vi "DB_Execute_Query.vi"() -> ()   [LabVIEW 2020]
uses:
  <vilib>/addons/database/Connection.llb/DB Tools Open Connec (String).vi
  <vilib>/addons/database/Connection.llb/Conn Execute.vi
  <vilib>/addons/database/Recordset.llb/Rec Fetch Recordset Data (R).vi
  <vilib>/addons/database/Recordset.llb/Rec Destroy - Connection.vi
  <vilib>/addons/database/NI_Database_API.lvlib
panel:
  out "recordset data":variant[][](array[variant])
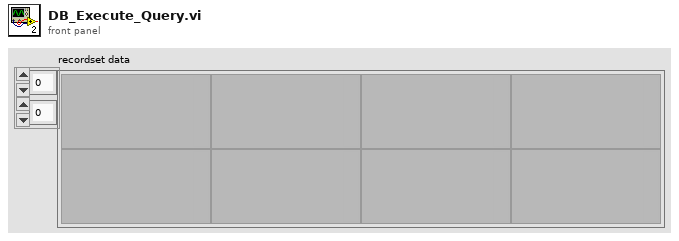
[diagram p1: front panel]
types:
  T1 = typedef "NI_Database_API.lvlib/Conn ObjectReference.ctl" = refnum<k1>
  T2 = typedef "NI_Database_API.lvlib/Rec ObjectReference.ctl" = refnum<k1>
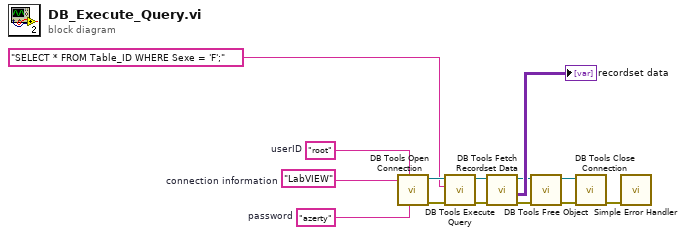
[diagram p0: block diagram]
diagram:
  w2 = "azerty"  # password
  w3 = "root"  # userID
  w4 = "LabVIEW"  # connection information
  n1 = call-poly <vilib>:"DB Tools Open Connection.vi"("password"=w2, "userID"=w3, "connection information"=w4) -> ("error out"=w13:errorcluster, "connection reference"=w14:T1)  [unwired: 5 in]
  n2 = call-poly <vilib>:"DB Tools Execute Query.vi"("error in (no error)"=w13, "SQL query"="SELECT * FROM Table_ID WHERE Sexe = 'F';", "connection reference"=w14) -> ("error out"=w8:errorcluster, "recordset reference"=w7:T2)  [unwired: 5 in]
  n3 = call-poly <vilib>:"DB Tools Fetch Recordset Data.vi"("error in (no error)"=w8, "recordset reference"=w7) -> ("error out"=w5:errorcluster, "recordset data"=→"recordset data":variant[][], "recordset reference out"=w6:T2)  [unwired: 3 in]
  n4 = call-poly <vilib>:"DB Tools Free Object.vi"("error in (no error)"=w5, "recordset reference"=w6) -> ("error out"=w10:errorcluster, "connection reference"=w12:T1)  [unwired: 8 in]
  n5 = call <vilib>:"DB Tools Close Connection.vi"("error in (no error)"=w10, "connection reference"=w12) -> ("error out"=w11:errorcluster)  [unwired: 5 in]
  n6 = call <vilib>:"Simple Error Handler.vi"("error in (no error)"=w11) -> ()  [unwired: 4 in, 5 out]
